vi "Capture@CalibrateManual__Parameter.vi"(1 "ParamterIn":string) -> (0 "ParamterOut":string)   [LabVIEW 2019]
uses:
  MainFrame/Global.vi
panel:
  out "Image":T1(plugin-control)
  in  "Picture":string(combo)
  in  "CamName":string(combo)
  in  "Confirm":bool
  # "Capture@General $Capture,$Picture"
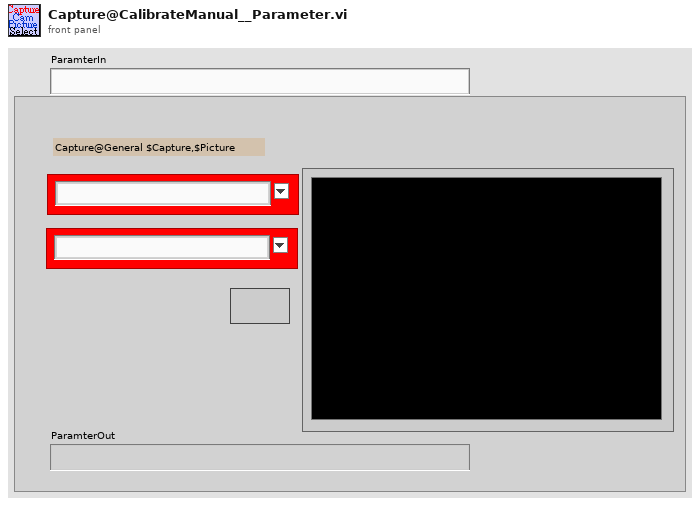
[diagram p1: front panel]
types:
  T1 = typedef "IMAQ Image.ctl" = refnum<image>
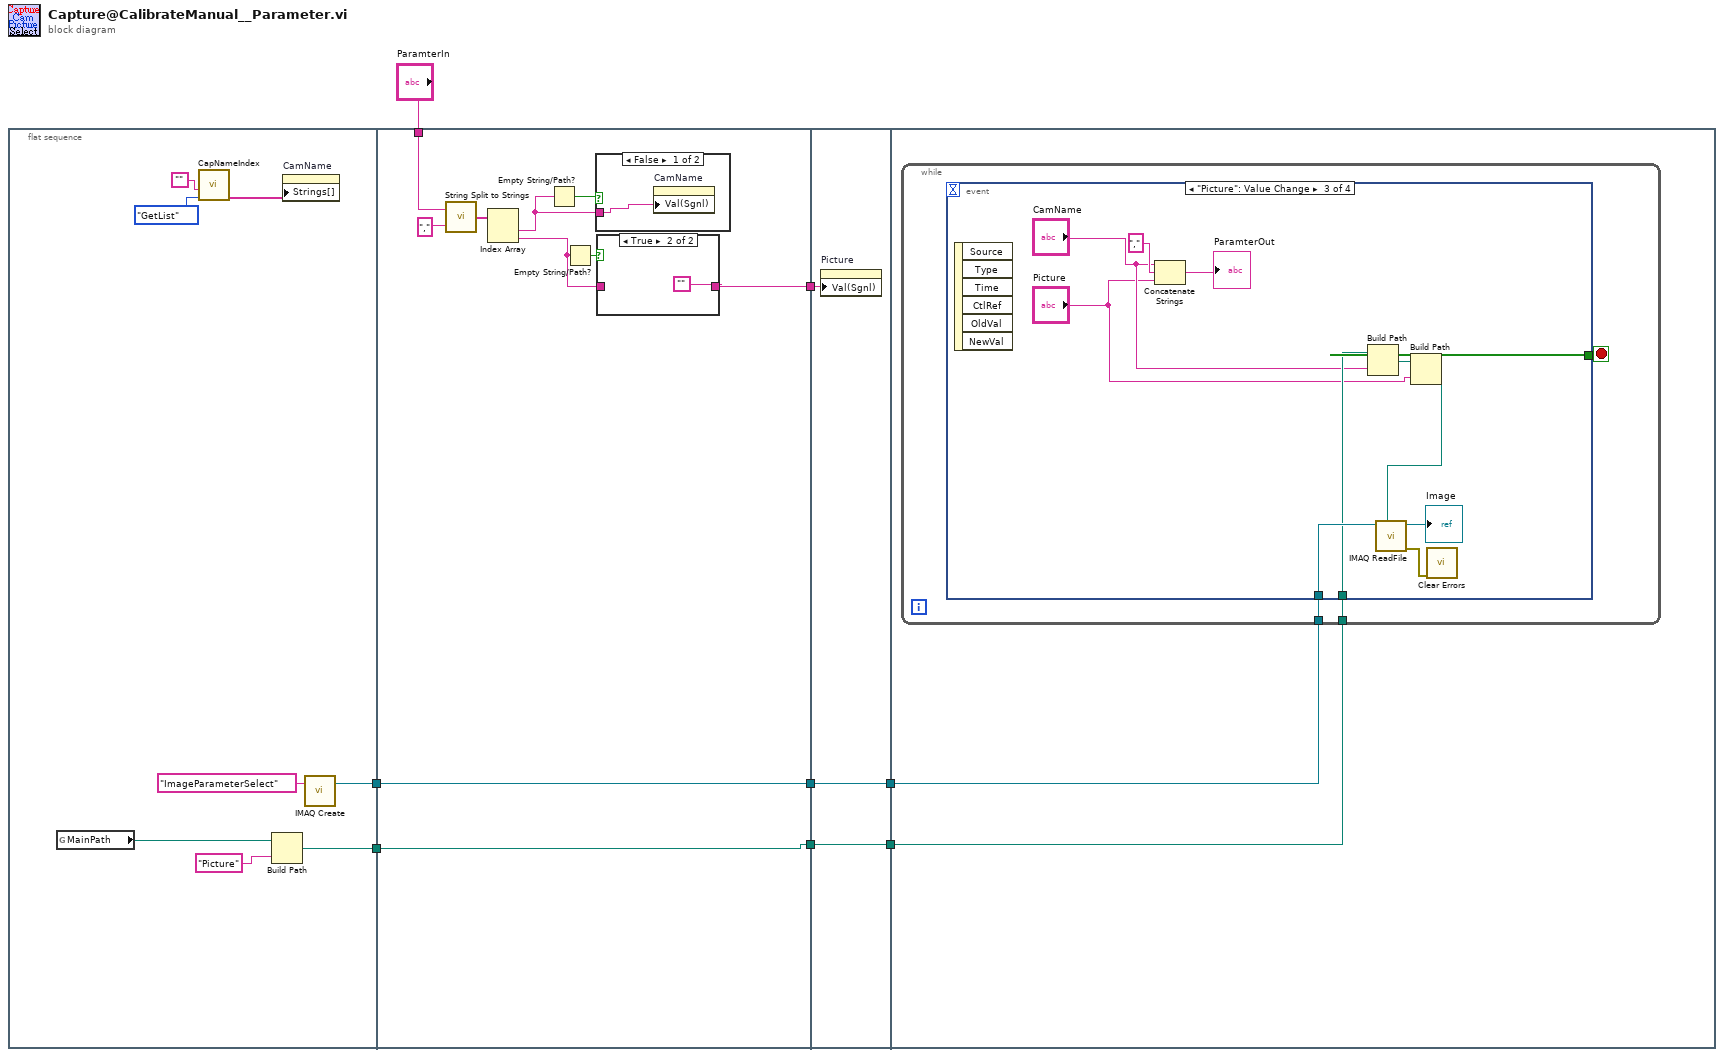
[diagram p0: block diagram]
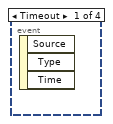
[diagram p4: hidden frame]
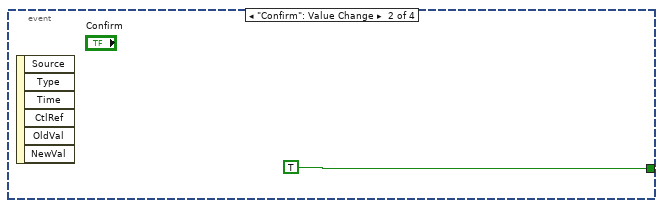
[diagram p5: hidden frame]
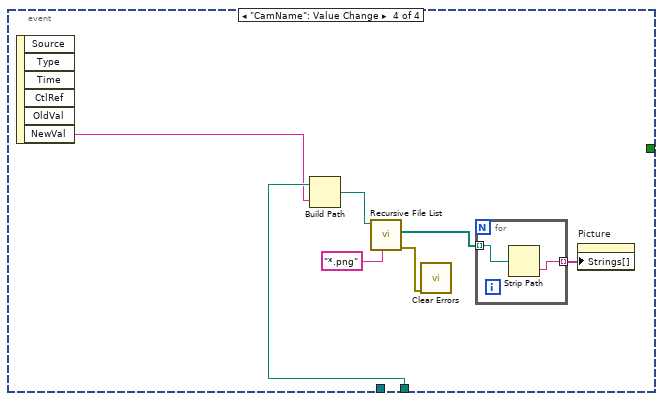
[diagram p6: hidden frame]
diagram:
  n1 = flat-sequence {
    tunnel: [w12] -> w7
    tunnel: [w10] -> w2
    tunnel: "ParamterIn" -> [w24]
    tunnel: w7 -> [w20]
    tunnel: [w20] -> w6
    tunnel: [w18] -> w3
    tunnel: w2 -> [w18]
    tunnel: [w17] -> w1
    tunnel: w6 -> [w32]
    tunnel: [w32] -> w5
    tunnel: [w31] -> w4
    tunnel: w3 -> [w31]
    tunnel: w1 -> [w30]
    tunnel: w5 -> [w34]
    tunnel: w4 -> [w33]
    frame #0 {
      n2 = global read "Global.vi" "MainPath"() -> (w9:path)
      n3 = call "CapNameIndex.vi"("OP"=enum16{"AddCam", "GetIndex", "Init", "GetList"}."GetList", "CamName"="") -> ("DeviceList"=w15:string[])  [unwired: 2 in, 3 out]
      n4 = Build Path(base path=w9, name or relative path="Picture") -> (appended path=w10:path)
      n5 = property on="CamName" class="CmbBox"("Strings[]"=w15) -> ()  [unwired: 2 in, 2 out]
      n6 = call "IMAQ Create"("Image Name"="ImageParameterSelect") -> ("New Image"=w12:T1)  [unwired: 4 in, 1 out]
    }
    frame #1 {
      n7 = call "String Split to Strings.vi"("search string/char (-)"=",", "String"=w24) -> ("Array"=w26:string[])
      n8 = Index Array(array=w26) -> (element #1=w19:string, element #2=w21:string)  [unwired: 2 in]
      n9 = Empty String/Path?(string/path=w19) -> (empty?=w23:bool)
      n10 = Empty String/Path?(string/path=w21) -> (empty?=w22:bool)
      n11 = case shown="False" w23 {
        tunnel: w19 -> [w29 _]
        frame False {
          n12 = property on="CamName" class="CmbBox"("Val(Sgnl)"=w29) -> ()  [unwired: 2 in, 2 out]
        }
        frame True {
        }
      }
      n13 = case shown="True" w22 {
        tunnel: [w27 ""] -> w17
        tunnel: w21 -> [w27 _]
        frame False {
        }
        frame True {
        }
      }
    }
    frame #2 {
      n14 = property on="Picture" class="CmbBox"("Val(Sgnl)"=w30) -> ()  [unwired: 2 in, 2 out]
    }
    frame #3 {
      n15 = while {
        tunnel: w34 -> [w36]
        tunnel: w33 -> [w35]
        stop <- w37 stop-if-true
        n16 = event shown="[2] \"Picture\": Value Change" {
          selector: _ -> [_ _ _ _]
          dyn-events: _ -> [_ _ _ _]
          timeout: _ -> [_ _ _ _]
          tunnel: [_ TRUE _ _] -> w37
          tunnel: w36 -> [_ _ w46 _]
          tunnel: w35 -> [_ _ w45 w52]
          event Timeout {
            n17 = event-data() -> ()  [unwired: 1 in, 3 out]
          }
          event "Confirm": Value Change {
            n18 = event-data() -> ()  [unwired: 1 in, 6 out]
          }
          event "Picture": Value Change {
            n19 = event-data() -> ()  [unwired: 1 in, 6 out]
            n20 = Concatenate Strings("CamName", "," ("string"), "Picture") -> (→"ParamterOut":string)
            n21 = Build Path(base path=w45, name or relative path="CamName") -> (appended path=w43:path)
            n22 = Build Path(base path=w43, name or relative path="Picture") -> (appended path=w41:path)
            n23 = call "IMAQ ReadFile"("File Path"=w41, "Image"=w46) -> ("error out"=w40:errorcluster, "Image Out"=→"Image":T1)  [unwired: 5 in, 3 out]
            n24 = call <vilib>:"Clear Errors.vi"("error in (no error)"=w40) -> ()  [unwired: 5 in, 2 out]
          }
          event "CamName": Value Change {
            n25 = event-data() -> ("NewVal"=w51:string)  [unwired: 1 in, 5 out]
            n26 = Build Path(base path=w52, name or relative path=w51) -> (appended path=w50:path)
            n27 = call <vilib>:"Recursive File List.vi"("pattern"="*.png", "Folder Path"=w50) -> ("error out"=w49:errorcluster, "All Files in Dir"=w54:path[])  [unwired: 5 in, 3 out]
            n28 = call <vilib>:"Clear Errors.vi"("error in (no error)"=w49) -> ()  [unwired: 5 in, 2 out]
            n29 = for {
              tunnel: w54 -> [w57] mode=indexing
              tunnel: [w56] -> w55 mode=indexing
              n30 = Strip Path(path=w57) -> (name=w56:string)  [unwired: 1 out]
            }
            n31 = property on="Picture" class="CmbBox"("Strings[]"=w55) -> ()  [unwired: 2 in, 2 out]
          }
        }
      }
    }
  }
